vi "GetSYSInfo.vi"(8 "error in (no error)":errorcluster) -> (0 "error out":errorcluster, 2 "Info":T1)   [LabVIEW 2020, in "ORM.lvlib" / "LogMap.lvclass"]
uses:
  LogMap.lvclass
  logmapcluster.ctl
  System.Management
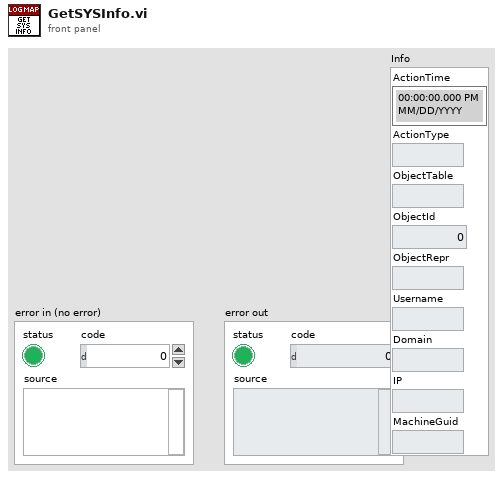
[diagram p1: front panel]
types:
  T1 = typedef "ORM.lvlib/LogMap.lvclass/logmapcluster.ctl" = cluster{"ActionTime":timestamp, "ActionType":string, "ObjectTable":string, "ObjectId":i64, "ObjectRepr":string, "Username":string, "Domain":string, "IP":string, "MachineGuid":string}
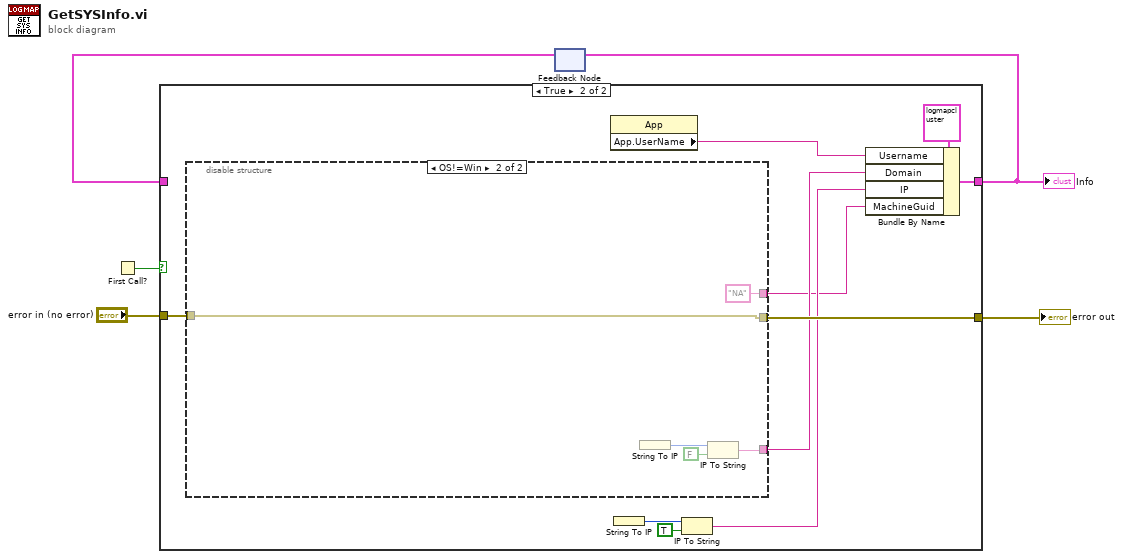
[diagram p0: block diagram]
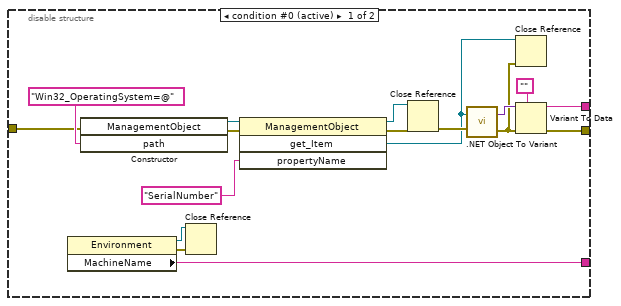
[diagram p3: hidden frame]
diagram:
  n1 = First Call?() -> (First Call?: T/F=w3:bool)
  n2 = feedback #1() -> (w1:T1)  [unwired: 1 in]
  n3 = case shown="True" w3 {
    tunnel: [w6 w16] -> w5
    tunnel: "error in (no error)" -> [w6 w15]
    tunnel: [w7 w10] -> w2
    tunnel: w1 -> [w7 _]
    frame False {
    }
    frame True {
      n4 = disable-structure shown="OS!=Win" {
        disable-tunnel: [w32 w35] -> w16
        disable-tunnel: w15 -> [w25 w35]
        disable-tunnel: [w24 w36] -> w13
        disable-tunnel: [w23 "NA"] -> w11
        frame condition #0 (active) {
          n5 = property class="Environment"() -> (reference out=w34:refnum<k24>, error out=w33:errorcluster, "MachineName"=w24:string)  [unwired: 2 in]
          n6 = constructor class="ManagementObject"(error in=w25, "path"="Win32_OperatingSystem=@") -> (reference out=w30:refnum<k24>, error out=w31:errorcluster)  [unwired: 2 in, 2 out]
          n7 = Close Reference(reference=w34, error in (no error)=w33) -> ()  [unwired: 1 out]
          n8 = invoke class="ManagementObject" method="get_Item"(reference=w30, error in=w31, "propertyName"="SerialNumber") -> (reference out=w20:refnum<k24>, error out=w22:errorcluster, "get_Item"=w19:refnum<k24>)  [unwired: 1 in, 1 out]
          n9 = Close Reference(reference=w20, error in (no error)=w22) -> (error out=w21:errorcluster)
          n10 = call <vilib>:".NET Object To Variant.vi"("error in (no error)"=w21, ".NET object"=w19) -> ("error out"=w18:errorcluster, "variant"=w27:variant)
          n11 = Close Reference(reference=w19, error in (no error)=w18) -> ()  [unwired: 1 out]
          n12 = Variant To Data(error in=w18, type="", Variant=w27) -> (data=w23:string, error out=w32:errorcluster)
        }
        frame condition #1 {
          n13 = String To IP() -> (0:w38:u32)  [unwired: 1 in]
          n14 = IP To String(1:FALSE ("dot notation? (F)"), 2:w38) -> (0:w36:string)
        }
      }
      n15 = property class="App"() -> ("App.UserName"=w8:string)  [unwired: 2 in, 2 out]
      n16 = String To IP() -> (0:w9:u32)  [unwired: 1 in]
      n17 = IP To String(1:TRUE ("dot notation? (F)"), 2:w9) -> (0:w12:string)
      n18 = Bundle By Name(cluster=T1 {"ActionTime"=timestamp(0 s since 1904-01-01), "ActionType"="", "ObjectTable"="", "ObjectId"=0, "ObjectRepr"="", "Username"="", "Domain"="", "IP"="", "MachineGuid"=""} ("Cluster of class private data"), "Username"=w8, "Domain"=w13, "IP"=w12, "MachineGuid"=w11) -> (w10:T1)
    }
  }
  "error out" <- w5
  "Info" <- w2
  n19 = feedback-in #1(w2) -> ()
